vi "Get Path Regex.vi"(8 "error in (no error)":errorcluster, 11 "ConnectRouteController in":refnum<class "ConnectRouteController.lvclass">) -> (0 "error out":errorcluster, 2 "Path Regex":string, 3 "ConnectRouteController out":refnum<class "ConnectRouteController.lvclass">)   [LabVIEW 2022 SP3, in "VideoMux.lvlib" / "ConnectRouteController.lvclass"]
uses:
  ConnectRouteController.lvclass
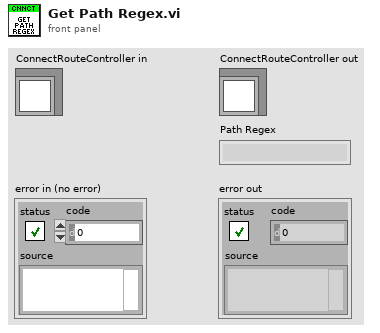
[diagram p1: front panel]
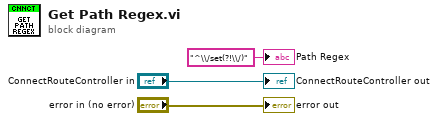
[diagram p0: block diagram]
diagram:
  "error out" <- "error in (no error)"
  "ConnectRouteController out" <- "ConnectRouteController in"
  "Path Regex" <- "^\\/set(?!\\/)" ("Path Regex")
